vi "Configure Trigger (AUDIO).vi"(0 "VISA resource name":refnum<visa-resource-name>, 5 "Trigger Source (9: Bus 1)":u16(ring)=9 items=["Bus 1"=9, "Bus 2"=10, "Bus 3"=11, "Bus 4"=12], 7 "Condition (0: Start of Frame)":u16(ring) items=["Start of Frame", "Data"], 9 "Data":T1={"Data Offset (0)"=0, "Data Upper Word Value (XXXXXXXX)"="XXXXXXXX", "Data Lower Word Value (XXXXXXXX)"="XXXXXXXX", "Data Qualifier (0: Less than)"=0, "Word Alignment (0: Either)"=0} {"Word Alignment (0: Either)" items=["Either", "Left", "Right"]; "Data Qualifier (0: Less than)" items=["Less than", "More than", "Equal", "Unequal", "Less equal", "More equal", "In range", "Out of range"]}, 11 "error in (no error)":errorcluster) -> (4 "VISA resource name out":refnum<visa-resource-name>, 15 "error out":errorcluster)   [LabVIEW 2013, in "Tektronix DPO MSO 2000 4000 Series.lvlib"]
doc: "Configures Audio trigger settings for an oscilloscope."
uses:
  Tektronix DPO MSO 2000 4000 Series.lvlib
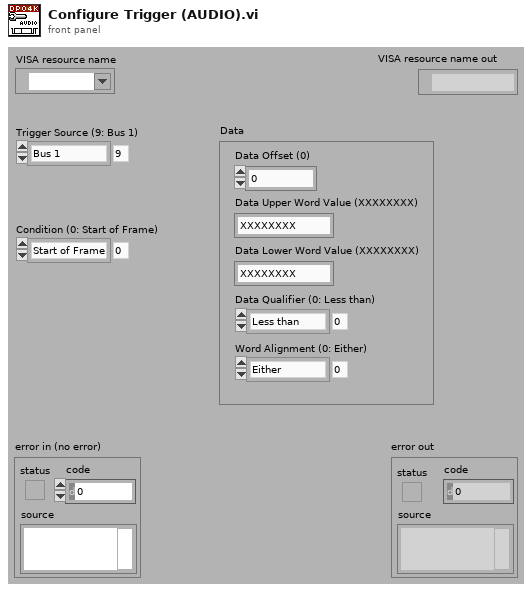
[diagram p1: front panel]
types:
  T1 = cluster{"Data Offset (0)":i32, "Data Upper Word Value (XXXXXXXX)":string, "Data Lower Word Value (XXXXXXXX)":string, "Data Qualifier (0: Less than)":u16, "Word Alignment (0: Either)":u16}
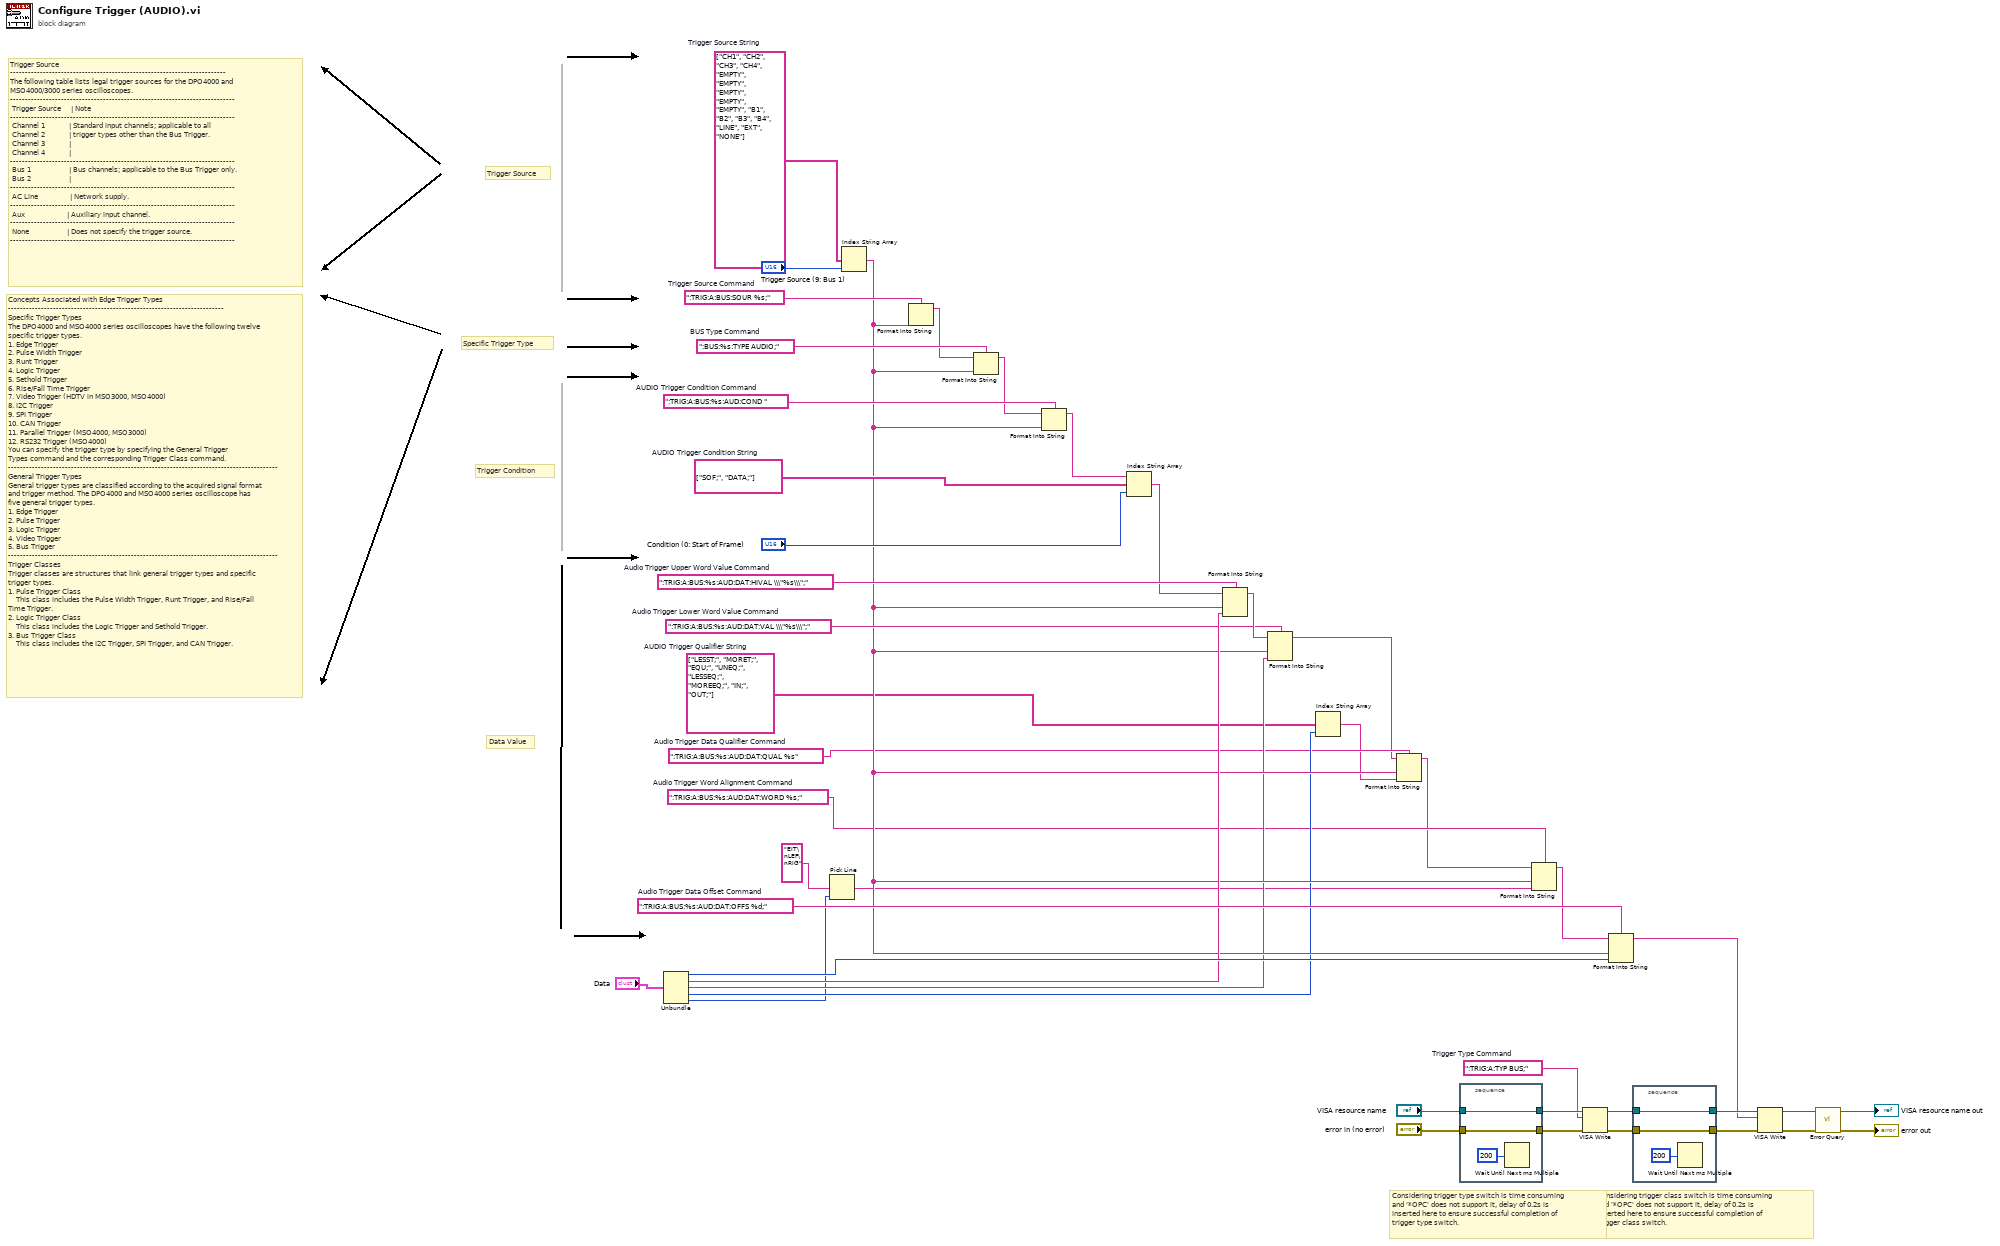
[diagram p0: block diagram]
diagram:
  w4 = ":TRIG:A:BUS:%s:AUD:DAT:WORD %s;"  # Audio Trigger Word Alignment Command
  w9 = ":TRIG:A:BUS:%s:AUD:DAT:QUAL %s"  # Audio Trigger Data Qualifier Command
  w11 = string[] ["LESST;", "MORET;", "EQU;", "UNEQ;", "LESSEQ;", "MOREEQ;", "IN;", "OUT;"]  # AUDIO Trigger Qualifier String
  w14 = ":TRIG:A:BUS:%s:AUD:DAT:VAL \\\"%s\\\";"  # Audio Trigger Lower Word Value Command
  w26 = string[] ["CH1", "CH2", "CH3", "CH4", "EMPTY", "EMPTY", "EMPTY", "EMPTY", "EMPTY", "B1", "B2", "B3", "B4", "LINE", "EXT", "NONE"]  # Trigger Source String
  w25 = ":TRIG:A:BUS:SOUR %s;"  # Trigger Source Command
  w33 = ":TRIG:A:TYP BUS;"  # Trigger Type Command
  w39 = ":TRIG:A:BUS:%s:AUD:DAT:OFFS %d;"  # Audio Trigger Data Offset Command
  w40 = ":TRIG:A:BUS:%s:AUD:DAT:HIVAL \\\"%s\\\";"  # Audio Trigger Upper Word Value Command
  w42 = string[] ["SOF;", "DATA;"]  # AUDIO Trigger Condition String
  w44 = ":TRIG:A:BUS:%s:AUD:COND "  # AUDIO Trigger Condition Command
  w24 = ":BUS:%s:TYPE AUDIO;"  # BUS Type Command
  # "Concepts Associated with Edge Trigger Types\n------------------------------------------------------------------------\nSpecific Trigger Types\nThe DPO4000 and MSO4000 series oscilloscopes have the following twelve specific trigger types.\n1. Edge Trigger\n2. Pulse Width Trigger\n3. Runt Trigger\n4. Logic Trigger\n5. Sethold Trigger\n6. Rise/Fall Time Trigger\n7. Video Trigger (HDTV in MSO3000, MSO4000)\n8. I2C Trigger\n9. SPI Trigger\n10. CAN Trigger\n11. Parallel Trigger (MSO4000, MSO3000)\n12. RS232 Trigger (MSO4000)\nYou can specify the trigger type by specifying the General Trigger \nTypes command and the corresponding Trigger Class command.\n------------------------------------------------------------------------------------------\nGeneral Trigger Types \nGeneral trigger types are classified according to the acquired signal format and trigger method. The DPO4000 and MSO4000 series oscilloscope has five general trigger types.\n1. Edge Trigger\n2. Pulse Trigger\n3. Logic Trigger\n4. Video Trigger\n5. Bus Trigger\n------------------------------------------------------------------------------------------\nTrigger Classes\nTrigger classes are structures that link general trigger types and specific trigger types.\n1. Pulse Trigger Class\n    This class includes the Pulse Width Trigger, Runt Trigger, and Rise/Fall Time Trigger.\n2. Logic Trigger Class\n    This class includes the Logic Trigger and Sethold Trigger.\n3. Bus Trigger Class\n    This class includes the I2C Trigger, SPI Trigger, and CAN Trigger."
  # "Trigger Source\n------------------------------------------------------------------------\nThe following table lists legal trigger sources for the DPO4000 and MSO4000/3000 series oscilloscopes.\n---------------------------------------------------------------------------\n Trigger Source     | Note                                                           \n---------------------------------------------------------------------------\n Channel 1            | Standard input channels; applicable to all      \n Channel 2            | trigger types other than the Bus Trigger.         \n Channel 3            |     \n Channel 4            |\n---------------------------------------------------------------------------\n Bus 1                   | Bus channels; applicable to the Bus Trigger only.\n Bus 2                   | \n---------------------------------------------------------------------------\n AC Line                | Network supply.\n---------------------------------------------------------------------------\n Aux                     | Auxiliary input channel.\n---------------------------------------------------------------------------\n None                   | Does not specify the trigger source.\n---------------------------------------------------------------------------"
  # "Data Value"
  # "Trigger Condition"
  # "Specific Trigger Type"
  # "Trigger Source"
  # "Considering trigger class switch is time consuming\nand '*OPC' does not support it, delay of 0.2s is \ninserted here to ensure successful completion of\ntrigger class switch."
  # "Considering trigger type switch is time consuming\nand '*OPC' does not support it, delay of 0.2s is \ninserted here to ensure successful completion of\ntrigger type switch."
  n1 = Unbundle("Data") -> ("Data Offset (0)"=w36:i32, "Data Upper Word Value (XXXXXXXX)"=w16:string, "Data Lower Word Value (XXXXXXXX)"=w12:string, "Data Qualifier (0: Less than)"=w10:u16, "Word Alignment (0: Either)"=w5:u16)
  n2 = Pick Line(multi-line string="EIT\nLEF\nRIG", line index=w5) -> (output string=w3:string)  [unwired: 1 in]
  n3 = Index String Array(1:"Trigger Source (9: Bus 1)", 2:w26) -> (0:w13:string)  [unwired: 1 in]
  n4 = Format Into String(format string=w25, w13) -> (resulting string=w21:string)  [unwired: 2 in, 1 out]
  n5 = Format Into String(format string=w24, initial string=w21, w13) -> (resulting string=w23:string)  [unwired: 1 in, 1 out]
  n6 = Format Into String(format string=w44, initial string=w23, w13) -> (resulting string=w43:string)  [unwired: 1 in, 1 out]
  n7 = Index String Array(1:"Condition (0: Start of Frame)", 2:w42, 3:w43) -> (0:w22:string)
  n8 = Format Into String(format string=w40, initial string=w22, w13, w16) -> (resulting string=w15:string)  [unwired: 1 in, 1 out]
  n9 = Format Into String(format string=w14, initial string=w15, w13, w12) -> (resulting string=w7:string)  [unwired: 1 in, 1 out]
  n10 = Index String Array(1:w10, 2:w11) -> (0:w8:string)  [unwired: 1 in]
  n11 = Format Into String(format string=w9, initial string=w7, w13, w8) -> (resulting string=w1:string)  [unwired: 1 in, 1 out]
  n12 = stacked-sequence {
    tunnel: "VISA resource name" -> [w47]
    tunnel: [w47] -> w35
    tunnel: "error in (no error)" -> [w46]
    tunnel: [w46] -> w34
    frame #0 {
      n13 = Wait Until Next ms Multiple(millisecond multiple=u32 200) -> ()  [unwired: 1 out]
    }
  }
  n14 = Format Into String(format string=w4, initial string=w1, w13, w3) -> (resulting string=w38:string)  [unwired: 1 in, 1 out]
  n15 = VISA Write(VISA resource name=w35, write buffer=w33, error in (no error)=w34) -> (VISA resource name out=w32:refnum<visa-resource-name>, error out=w31:errorcluster)  [unwired: 1 out]
  n16 = Format Into String(format string=w39, initial string=w38, w13, w36) -> (resulting string=w2:string)  [unwired: 1 in, 1 out]
  n17 = stacked-sequence {
    tunnel: w32 -> [w50]
    tunnel: [w50] -> w27
    tunnel: w31 -> [w49]
    tunnel: [w49] -> w30
    frame #0 {
      n18 = Wait Until Next ms Multiple(millisecond multiple=u32 200) -> ()  [unwired: 1 out]
    }
  }
  n19 = VISA Write(VISA resource name=w27, write buffer=w2, error in (no error)=w30) -> (VISA resource name out=w29:refnum<visa-resource-name>, error out=w28:errorcluster)  [unwired: 1 out]
  n20 = call "Error Query.vi"("error in (no error)"=w28, "VISA resource name"=w29) -> ("error out"=→"error out":errorcluster, "VISA resource name out"=→"VISA resource name out":refnum<visa-resource-name>)  [unwired: 6 in, 2 out]
